vi "全局 数据发送重叠.vi"() -> ()   [LabVIEW 2016]
panel:
  out "数据发送重叠开始时间戳":string
  out "数据发送重叠":bool
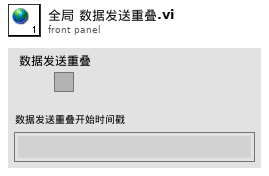
[diagram p1: front panel]
diagram:
